vi "Error LOG.vi"(0 "Error Handler in":refnum<class "TLB` Error Handler.lvclass">, 5 "action queue in":refnum<queue>, 7 "log action":T1, 11 "addtional error information":string) -> (4 "Error Handler out":refnum<class "TLB` Error Handler.lvclass">, 15 "error out":errorcluster)   [LabVIEW 2015, in "TLB` Template.lvlib" / "TLB` Error Handler.lvclass"]
doc: "insert <B>log</B> into action queue.\n\n<B>Input Parameters</B>\n\n<B>Error Handler in</B> identifies your session. <B>Error Handler in</B> is obtained from the Open.vi of this class.\n\n<B>action queue in</B> is a reference to a queue. Use the Create Action Queue function to obtain a queue reference. \n\n<B>error action</B>\n<B>Default</B> functionality.\n<B>Override</B> the default functionality.\n<B>Append to Beginning</B> in addition to default functionality.\n<B>Append to End</B> in addition to default functionality.\n\n<B>additional error information</B> to be inserted into the error log file.\n\n<B>Output Parameters</B>\n\n<B>Error Handler out</B> identifies your session. 'Error Handler out' is obtained from the Open.vi of this class.\n\n<B>error out</B> contains error information. This output provides standard error out functionality."
uses:
  TLB` Error Handler.lvclass
  Actions/Actions.lvlib
  Actions/System Action Element.ctl
  typedef/Log Action.ctl
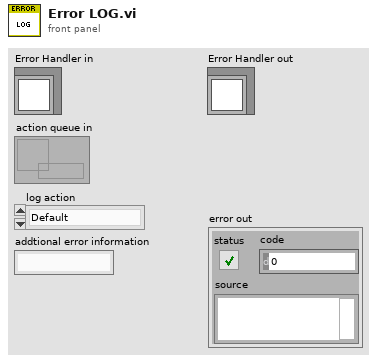
[diagram p1: front panel]
types:
  T1 = typedef "TLB` Template.lvlib/TLB` Error Handler.lvclass/Log Action.ctl" = enum16{"Default", "Override", "Appended to Beginning", "Append to End"}
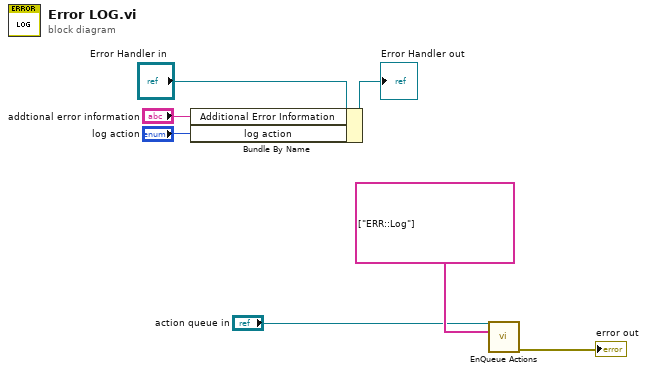
[diagram p0: block diagram]
diagram:
  n1 = Bundle By Name(cluster="Error Handler in", "Additional Error Information"="addtional error information", "log action"="log action") -> (→"Error Handler out":refnum<class "TLB` Error Handler.lvclass">)
  n2 = call "EnQueue Actions.vi"("action queue in"="action queue in", "actions"=string[] ["ERR::Log"] ("message names")) -> ("error out"=→"error out":errorcluster)  [unwired: 12 in, 1 out]
